vi "GyroErrorCompensation.vi"(4 "error in":errorcluster, 5 "Angular Rate":dbl format="%#_13g", 6 "Angle":dbl format="%#_13g") -> (0 "error out":errorcluster, 2 "Virtual Angle":dbl)   [LabVIEW 2016]
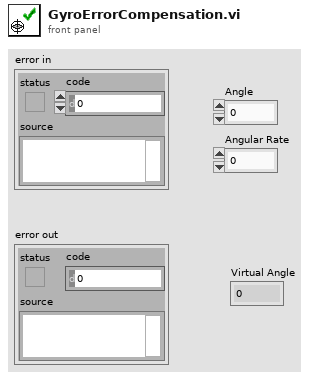
[diagram p1: front panel]
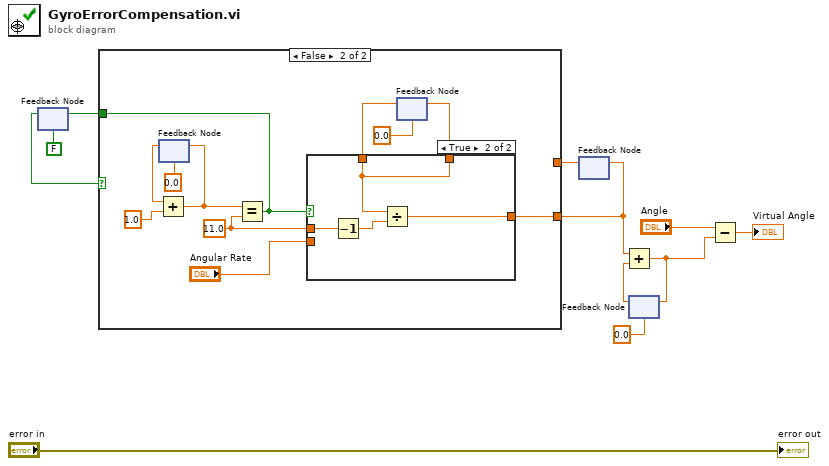
[diagram p0: block diagram]
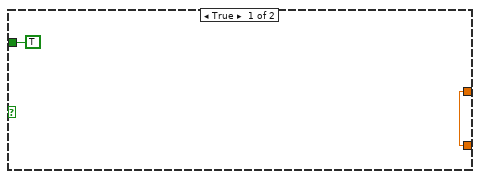
[diagram p2: hidden frame]
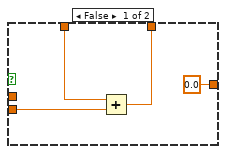
[diagram p3: hidden frame]
diagram:
  n1 = feedback #1(FALSE) -> (w5:bool)
  n2 = feedback #2() -> (w3:dbl)  [unwired: 1 in]
  n3 = case shown="False" w5 {
    tunnel: [w13 w15] -> w4
    tunnel: [TRUE w14] -> w6
    tunnel: w3 -> [w13 _]
    frame True {
    }
    frame False {
      w16 = 11.0 ("y")
      n4 = feedback #3(0.0) -> (w21:dbl)
      n5 = Add(x=w21, y=1.0) -> (x+y=w23:dbl)
      n6 = feedback-in #3(w23) -> ()
      n7 = Equal?(x=w23, y=w16) -> (x = y?=w14:bool)
      n8 = feedback #4(0.0) -> (w18:dbl)
      n9 = case shown="True" w14 {
        tunnel: "Angular Rate" -> [w28 _]
        tunnel: [w27 w29] -> w19
        tunnel: w18 -> [w26 w29]
        tunnel: w16 -> [_ w32]
        tunnel: [0.0 w30] -> w15
        frame False {
          n10 = Add(x=w26, y=w28) -> (x+y=w27:dbl)
        }
        frame True {
          n11 = Decrement(x=w32) -> (x-1=w31:dbl)
          n12 = Divide(x=w29, y=w31) -> (x/y=w30:dbl)
        }
      }
      n13 = feedback-in #4(w19) -> ()
    }
  }
  n14 = feedback-in #1(w6) -> ()
  n15 = feedback-in #2(w4) -> ()
  n16 = feedback #5(0.0) -> (w10:dbl)
  n17 = Add(x=w4, y=w10) -> (x+y=w8:dbl)
  n18 = feedback-in #5(w8) -> ()
  n19 = Subtract(x="Angle", y=w8) -> (x-y=→"Virtual Angle":dbl)
  "error out" <- "error in"
